vi "workbook set properties.vi"(8 "error in (no error)":errorcluster, 10 "properties":u32, 11 "workbook":u32) -> (0 "error out":errorcluster, 3 "function return":u32(ring))   [LabVIEW 8.6]
doc: "lxw_error workbook_set_properties(lxw_workbook workbook, unsigned long properties);"
uses:
  pending_lvxlsxwriter/xlsxwriter.dll
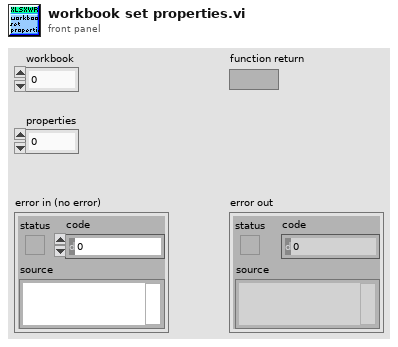
[diagram p1: front panel]
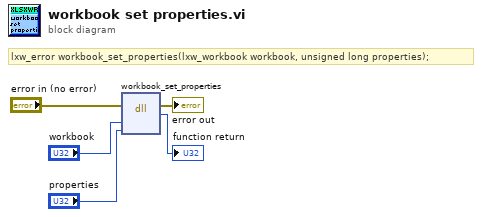
[diagram p0: block diagram]
diagram:
  # "lxw_error workbook_set_properties(lxw_workbook workbook, unsigned long properties);"
  n1 = dll-call lib="C:/Users/WDAGUtilityAccount/Desktop/pending_lvxlsxwriter/xlsxwriter.*" fn="workbook_set_properties"(error in="error in (no error)", "workbook"="workbook", "properties"="properties") -> (error out=→"error out":errorcluster, →"function return":u32)  [unwired: 4 in, 1 out]
